vi "BRig_dataExp_CueSwitch_Prob_First.vi"() -> (2 "output_CueSwitch_Prob_First":i32)   [LabVIEW 2014]
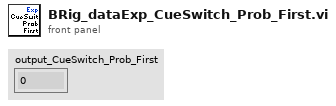
[diagram p1: front panel]
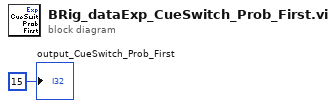
[diagram p0: block diagram]
diagram:
  "output_CueSwitch_Prob_First" <- 15 ("output_iBlock")
